vi "Overlay Image.vi"(7 "overlay images":T1[](array[typedef]), 8 "error in":errorcluster, 9 "image name in":string, 10 "overlay":T2, 11 "path in":path) -> (0 "error out":errorcluster, 2 "overlayed image name":string, 3 "image data":T1)   [LabVIEW 2013, in "configuration library.lvlib"]
uses:
  configuration library.lvlib
  <vilib>/NI/Tag Bus Data Framework/Configuration Editor/subVIs/Glyphs Status.ctl
  <vilib>/picture/picture.llb/imagedata.ctl
  <vilib>/NI/Tag Bus Data Framework/Configuration Editor/PL Framework Configuration Tool.lvlib
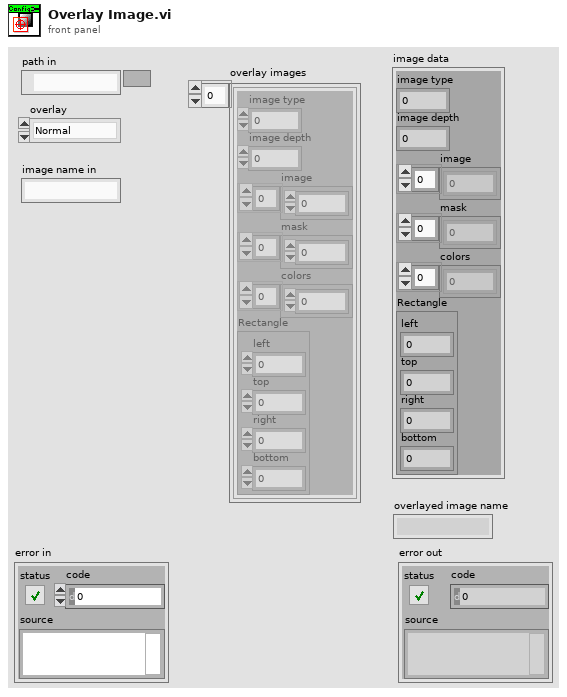
[diagram p1: front panel]
types:
  T1 = typedef "imagedata.ctl" = cluster{"image type":i32, "image depth":i32, "image":u8[], "mask":u8[], "colors":u32[], "Rectangle":cluster{"left":i16, "top":i16, "right":i16, "bottom":i16}}
  T2 = typedef "PL Framework Configuration Tool.lvlib/Glyphs Status.ctl" = enum16{"Normal", "Error"}
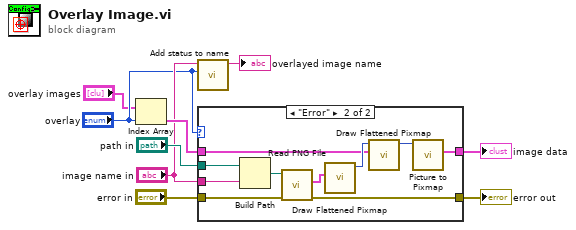
[diagram p0: block diagram]
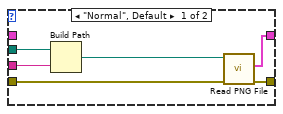
[diagram p2: hidden frame]
diagram:
  n1 = Index Array(array="overlay images", index="overlay") -> (element=w5:T1)
  n2 = call <vilib>:"Add status to name.vi"("Status"="overlay", "Name"="image name in") -> ("Name with status"=→"overlayed image name":string)  [unwired: 9 in]
  n3 = case shown="\"Error\"" "overlay" {
    tunnel: "path in" -> [w15 w20]
    tunnel: [w13 w22] -> w9
    tunnel: "image name in" -> [w12 w19]
    tunnel: "error in" -> [w11 w18]
    tunnel: [w10 w17] -> w6
    tunnel: w5 -> [_ w16]
    frame "Normal", Default {
      n4 = Build Path(base path=w15, name or relative path=w12) -> (appended path=w14:path)
      n5 = call <vilib>:"Read PNG File.vi"("error in (no error)"=w11, "path to PNG file"=w14) -> ("error out"=w10:errorcluster, "image data"=w13:T1)  [unwired: 7 in, 1 out]
    }
    frame "Error" {
      n6 = Build Path(base path=w20, name or relative path=w19) -> (appended path=w25:path)
      n7 = call <vilib>:"Read PNG File.vi"("error in (no error)"=w18, "path to PNG file"=w25) -> ("error out"=w17:errorcluster, "image data"=w23:T1)  [unwired: 7 in, 1 out]
      n8 = call <vilib>:"Draw Flattened Pixmap.vi"("image data"=w23) -> ("new picture"=w21:picture)  [unwired: 8 in]
      n9 = call <vilib>:"Draw Flattened Pixmap.vi"("image data"=w16, "picture"=w21) -> ("new picture"=w24:picture)  [unwired: 7 in]
      n10 = call <vilib>:"Picture to Pixmap.vi"("picture"=w24) -> ("image data"=w22:T1)  [unwired: 9 in, 1 out]
    }
  }
  "image data" <- w9
  "error out" <- w6
